vi "initialize StrainCell.vi"(9 "字符串":string, 11 "config in":T1={"initialize"=enum."SR830", "6221"={"6221 Resource"="GPIB1::10::INSTR", "Delta status"=FALSE, "电流|RMS(A)"=0.0}, "SR830+6221"={"source"=0, "Current(A)"=0.0, "阻抗(Ohm)"=0.0, "SR830 1"=FALSE, "SR830 2"=FALSE, "SR830 3"=FALSE, "SR830 4"=FALSE, "VISA 1"="GPIB1::1::INSTR", "VISA 2"="GPIB1::2::INSTR", "VISA 3"="GPIB1::3::INSTR", "VISA 4"="GPIB1::4::INSTR", "Reserve 1"=-1, "Reserve 2"=-1, "Reserve 3"=-1, "Reserve 4"=-1, "Sensitivity 1"=-1, "Sensitivity 2"=0, "Sensitivity 3"=-1, "Sensitivity 4"=-1, "量程入 1"=0, "量程入 2"=0, "量程入 3"=0, "量程入 4"=0}, "2400"={"2400"=FALSE, "VISA"="GPIB0::9::INSTR", "Output Level (0)"=1e-05, "Compliance  Level (0.1)"=10.0, "ch"=[1, 2, 1, 2]}, "ch"={"ch"=[], "current"=[], "change?"=[], "holding current\nwhen change ch?"=TRUE, "current offset"=[]}, "Instrument"={"limit"={"Field limit"=0.0, "Field rate limit"=0.0, "Temp limit"=0.0, "Temp low limit"=0.0, "Temp rate limit "=0.0}, "genarl"={"行数"=refnum, "编辑列表框？"=refnum, "列表框"=refnum, "camg 振荡状态"=refnum, "Aborting"=refnum, "数据文件"=refnum, "warning"=refnum, "vi路径"="", "Instrument Type"=enum."PPMS"}, "cmag"={"TM620"="TCPIP0::192.168.1.5::4266::SOCKET", "M24C Resource"="", "4G supply"="", "Temp Status 24C"=refnum, "Temp"=refnum, "9T信号"=refnum, "4g supply status"=refnum, "in-plane"="", "out-plane"="", "in-plane signal"=FALSE, "out-plane signal"=FALSE, "in plane 信号"=refnum, "pzt volt"=refnum, "camg Rate"=refnum}, "lengtou2"={"750 visa"="", "750 rotate"="", "semaphore 340"=refnum, "semaphore 750"=refnum, "750 field status"=refnum, "Input (0:A) 340"=0, "340 Resource"="GPIB0::14::INSTR", "340 Status"=refnum, "Input (0:B) 340"=0, "Loop (0: 1)"=0, "Loop (1: 1)"=0, "TCP master instance"=refnum}, "lengtou"={"TCP master instance"=refnum, "335 Status"=refnum, "335 Resource "="", "Input (0:A) 335"=0, "Input (0:B) 335"=0, "Heater Output (1:1) 335"=0, "semaphore 335"=refnum}, "325 for test"={"quantum design"=refnum, "semaphore 325"=refnum, "325 Resource "="", "Input (0:A) 325"=0, "Heater Output (1:1) 325"=0, "325 Status"=refnum}}, "2614B"={"2614B chA"=FALSE, "2614B chB"=FALSE, "VISA"="GPIB1::5::INSTR"}, "33522b"={"33522b resource name"="GPIB0::16::INSTR", "零电压"=0.0, "最大电压"=150.0, "间隔"=4.0, "最小电压"=-50.0, "loop"=2.0, "压电陶瓷电压(Vpp)"=0.0}, "gating type"=enum."2614(daul)", "层数"=0, "行数"=0, "是否处理"=[], "current 2"=[], "StrainCell"={"RP100 resource name"="GPIB0::16::INSTR", "E4980 resource name"="GPIB0::16::INSTR", "RP100 Reset ?(True)"=TRUE, "Voltage1(V)"=0.0, "Voltage2(V)"=0.0, "interval"=4.0, "slew(V/s)"=1.0}} {"Instrument"."325 for test"."Heater Output (1:1) 325" items=["1"=1, "2"=2]; "Instrument"."325 for test"."Input (0:A) 325" items=["A", "B"]; "Instrument"."lengtou"."Heater Output (1:1) 335" items=["1"=1, "2"=2]; "Instrument"."lengtou"."Input (0:B) 335" items=["A", "B"]; "Instrument"."lengtou"."Input (0:A) 335" items=["A", "B"]; "Instrument"."lengtou2"."Loop (1: 1)" items=["1", "2"]; "Instrument"."lengtou2"."Loop (0: 1)" items=["1", "2"]; "Instrument"."lengtou2"."Input (0:B) 340" items=["A", "B", "C", "D"]; "Instrument"."lengtou2"."Input (0:A) 340" items=["A", "B", "C", "D"]; "SR830+6221"."Sensitivity 4" items=["Auto Gain"=-1, "2 nV/fA"=0, "5 nV/fA"=1, "10 nV/fA"=2, "20 nV/fA"=3, "50 nV/fA"=4, "100 nV/fA"=5, "200 nV/fA"=6, "500 nV/fA"=7, "1 uV/pA"=8, "2 uV/pA"=9, "5 uV/pA"=10, "10 uV/pA"=11, "20 uV/pA"=12, "50 uV/pA"=13, "100 uV/pA"=14, "200 uV/pA"=15, "500 uV/pA"=16, "1 mV/nA"=17, "2 mV/nA"=18, "5 mV/nA"=19, "10 mV/nA"=20, "20 mV/nA"=21, "50 mV/nA"=22, "100 mV/nA"=23, "200 mV/nA"=24, "500 mV/mA"=25, "1 V/uA"=26]; "SR830+6221"."Sensitivity 3" items=["Auto Gain"=-1, "2 nV/fA"=0, "5 nV/fA"=1, "10 nV/fA"=2, "20 nV/fA"=3, "50 nV/fA"=4, "100 nV/fA"=5, "200 nV/fA"=6, "500 nV/fA"=7, "1 uV/pA"=8, "2 uV/pA"=9, "5 uV/pA"=10, "10 uV/pA"=11, "20 uV/pA"=12, "50 uV/pA"=13, "100 uV/pA"=14, "200 uV/pA"=15, "500 uV/pA"=16, "1 mV/nA"=17, "2 mV/nA"=18, "5 mV/nA"=19, "10 mV/nA"=20, "20 mV/nA"=21, "50 mV/nA"=22, "100 mV/nA"=23, "200 mV/nA"=24, "500 mV/mA"=25, "1 V/uA"=26]; "SR830+6221"."Sensitivity 1" items=["Auto Gain"=-1, "2 nV/fA"=0, "5 nV/fA"=1, "10 nV/fA"=2, "20 nV/fA"=3, "50 nV/fA"=4, "100 nV/fA"=5, "200 nV/fA"=6, "500 nV/fA"=7, "1 uV/pA"=8, "2 uV/pA"=9, "5 uV/pA"=10, "10 uV/pA"=11, "20 uV/pA"=12, "50 uV/pA"=13, "100 uV/pA"=14, "200 uV/pA"=15, "500 uV/pA"=16, "1 mV/nA"=17, "2 mV/nA"=18, "5 mV/nA"=19, "10 mV/nA"=20, "20 mV/nA"=21, "50 mV/nA"=22, "100 mV/nA"=23, "200 mV/nA"=24, "500 mV/mA"=25, "1 V/uA"=26]; "SR830+6221"."Sensitivity 2" items=["Auto Gain"=-1, "2 nV/fA"=0, "5 nV/fA"=1, "10 nV/fA"=2, "20 nV/fA"=3, "50 nV/fA"=4, "100 nV/fA"=5, "200 nV/fA"=6, "500 nV/fA"=7, "1 uV/pA"=8, "2 uV/pA"=9, "5 uV/pA"=10, "10 uV/pA"=11, "20 uV/pA"=12, "50 uV/pA"=13, "100 uV/pA"=14, "200 uV/pA"=15, "500 uV/pA"=16, "1 mV/nA"=17, "2 mV/nA"=18, "5 mV/nA"=19, "10 mV/nA"=20, "20 mV/nA"=21, "50 mV/nA"=22, "100 mV/nA"=23, "200 mV/nA"=24, "500 mV/mA"=25, "1 V/uA"=26]; "SR830+6221"."Reserve 4" items=["Auto Reserve"=-1, "High Reserve"=0, "Normal"=1, "Low Noise"=2]; "SR830+6221"."Reserve 3" items=["Auto Reserve"=-1, "High Reserve"=0, "Normal"=1, "Low Noise"=2]; "SR830+6221"."Reserve 2" items=["Auto Reserve"=-1, "High Reserve"=0, "Normal"=1, "Low Noise"=2]; "SR830+6221"."Reserve 1" items=["Auto Reserve"=-1, "High Reserve"=0, "Normal"=1, "Low Noise"=2]; "SR830+6221"."source" items=["SR830 1", "SR830 2", "SR830 3", "SR830 4"]}) -> (3 "输出簇":T1={"initialize"=enum."SR830", "6221"={"6221 Resource"="GPIB0::24::INSTR", "Delta status"=FALSE, "电流|RMS(A)"=0.0}, "SR830+6221"={"source"=0, "Current(A)"=0.0, "阻抗(Ohm)"=0.0, "SR830 1"=FALSE, "SR830 2"=FALSE, "SR830 3"=FALSE, "SR830 4"=FALSE, "VISA 1"="", "VISA 2"="", "VISA 3"="", "VISA 4"="", "Reserve 1"=-1, "Reserve 2"=-1, "Reserve 3"=-1, "Reserve 4"=-1, "Sensitivity 1"=-1, "Sensitivity 2"=-1, "Sensitivity 3"=-1, "Sensitivity 4"=-1, "量程入 1"=0, "量程入 2"=0, "量程入 3"=0, "量程入 4"=0}, "2400"={"2400"=FALSE, "VISA"="GPIB0::9::INSTR", "Output Level (0)"=1e-05, "Compliance  Level (0.1)"=10.0, "ch"=[]}, "ch"={"ch"=[], "current"=[], "change?"=[], "holding current\nwhen change ch?"=FALSE, "current offset"=[]}, "Instrument"={"limit"={"Field limit"=0.0, "Field rate limit"=0.0, "Temp limit"=0.0, "Temp low limit"=0.0, "Temp rate limit "=0.0}, "genarl"={"行数"=refnum, "编辑列表框？"=refnum, "列表框"=refnum, "camg 振荡状态"=refnum, "Aborting"=refnum, "数据文件"=refnum, "warning"=refnum, "vi路径"="", "Instrument Type"=enum."SVSM"}, "cmag"={"TM620"="GPIB0::24::INSTR", "M24C Resource"="GPIB0::24::INSTR", "4G supply"="GPIB0::24::INSTR", "Temp Status 24C"=refnum, "Temp"=refnum, "9T信号"=refnum, "4g supply status"=refnum, "in-plane"="", "out-plane"="", "in-plane signal"=TRUE, "out-plane signal"=FALSE, "in plane 信号"=refnum, "pzt volt"=refnum, "camg Rate"=refnum}, "lengtou2"={"750 visa"="", "750 rotate"="", "semaphore 340"=refnum, "semaphore 750"=refnum, "750 field status"=refnum, "Input (0:A) 340"=1, "340 Resource"="GPIB0::14::INSTR", "340 Status"=refnum, "Input (0:B) 340"=0, "Loop (0: 1)"=1, "Loop (1: 1)"=0, "TCP master instance"=refnum}, "lengtou"={"TCP master instance"=refnum, "335 Status"=refnum, "335 Resource "="GPIB0::24::INSTR", "Input (0:A) 335"=0, "Input (0:B) 335"=0, "Heater Output (1:1) 335"=0, "semaphore 335"=refnum}, "325 for test"={"quantum design"=refnum, "semaphore 325"=refnum, "325 Resource "="GPIB0::13::INSTR", "Input (0:A) 325"=1000, "Heater Output (1:1) 325"=1, "325 Status"=refnum}}, "2614B"={"2614B chA"=FALSE, "2614B chB"=FALSE, "VISA"=""}, "33522b"={"33522b resource name"="GPIB0::16::INSTR", "零电压"=0.0, "最大电压"=148.0, "间隔"=4.0, "最小电压"=-48.0, "loop"=3.0, "压电陶瓷电压(Vpp)"=0.0}, "gating type"=enum."2614(daul)", "层数"=0, "行数"=0, "是否处理"=[], "current 2"=[], "StrainCell"={"RP100 resource name"="GPIB0::16::INSTR", "E4980 resource name"="GPIB0::16::INSTR", "RP100 Reset ?(True)"=TRUE, "Voltage1(V)"=0.0, "Voltage2(V)"=148.0, "interval"=4.0, "slew(V/s)"=-48.0}} {"Instrument"."325 for test"."Heater Output (1:1) 325" items=["1"=1, "2"=2]; "Instrument"."325 for test"."Input (0:A) 325" items=["A", "B"]; "Instrument"."lengtou"."Heater Output (1:1) 335" items=["1"=1, "2"=2]; "Instrument"."lengtou"."Input (0:B) 335" items=["A", "B"]; "Instrument"."lengtou"."Input (0:A) 335" items=["A", "B"]; "Instrument"."lengtou2"."Loop (1: 1)" items=["1", "2"]; "Instrument"."lengtou2"."Loop (0: 1)" items=["1", "2"]; "Instrument"."lengtou2"."Input (0:B) 340" items=["A", "B", "C", "D"]; "Instrument"."lengtou2"."Input (0:A) 340" items=["A", "B", "C", "D"]; "SR830+6221"."Sensitivity 4" items=["Auto Gain"=-1, "2 nV/fA"=0, "5 nV/fA"=1, "10 nV/fA"=2, "20 nV/fA"=3, "50 nV/fA"=4, "100 nV/fA"=5, "200 nV/fA"=6, "500 nV/fA"=7, "1 uV/pA"=8, "2 uV/pA"=9, "5 uV/pA"=10, "10 uV/pA"=11, "20 uV/pA"=12, "50 uV/pA"=13, "100 uV/pA"=14, "200 uV/pA"=15, "500 uV/pA"=16, "1 mV/nA"=17, "2 mV/nA"=18, "5 mV/nA"=19, "10 mV/nA"=20, "20 mV/nA"=21, "50 mV/nA"=22, "100 mV/nA"=23, "200 mV/nA"=24, "500 mV/mA"=25, "1 V/uA"=26]; "SR830+6221"."Sensitivity 3" items=["Auto Gain"=-1, "2 nV/fA"=0, "5 nV/fA"=1, "10 nV/fA"=2, "20 nV/fA"=3, "50 nV/fA"=4, "100 nV/fA"=5, "200 nV/fA"=6, "500 nV/fA"=7, "1 uV/pA"=8, "2 uV/pA"=9, "5 uV/pA"=10, "10 uV/pA"=11, "20 uV/pA"=12, "50 uV/pA"=13, "100 uV/pA"=14, "200 uV/pA"=15, "500 uV/pA"=16, "1 mV/nA"=17, "2 mV/nA"=18, "5 mV/nA"=19, "10 mV/nA"=20, "20 mV/nA"=21, "50 mV/nA"=22, "100 mV/nA"=23, "200 mV/nA"=24, "500 mV/mA"=25, "1 V/uA"=26]; "SR830+6221"."Sensitivity 1" items=["Auto Gain"=-1, "2 nV/fA"=0, "5 nV/fA"=1, "10 nV/fA"=2, "20 nV/fA"=3, "50 nV/fA"=4, "100 nV/fA"=5, "200 nV/fA"=6, "500 nV/fA"=7, "1 uV/pA"=8, "2 uV/pA"=9, "5 uV/pA"=10, "10 uV/pA"=11, "20 uV/pA"=12, "50 uV/pA"=13, "100 uV/pA"=14, "200 uV/pA"=15, "500 uV/pA"=16, "1 mV/nA"=17, "2 mV/nA"=18, "5 mV/nA"=19, "10 mV/nA"=20, "20 mV/nA"=21, "50 mV/nA"=22, "100 mV/nA"=23, "200 mV/nA"=24, "500 mV/mA"=25, "1 V/uA"=26]; "SR830+6221"."Sensitivity 2" items=["Auto Gain"=-1, "2 nV/fA"=0, "5 nV/fA"=1, "10 nV/fA"=2, "20 nV/fA"=3, "50 nV/fA"=4, "100 nV/fA"=5, "200 nV/fA"=6, "500 nV/fA"=7, "1 uV/pA"=8, "2 uV/pA"=9, "5 uV/pA"=10, "10 uV/pA"=11, "20 uV/pA"=12, "50 uV/pA"=13, "100 uV/pA"=14, "200 uV/pA"=15, "500 uV/pA"=16, "1 mV/nA"=17, "2 mV/nA"=18, "5 mV/nA"=19, "10 mV/nA"=20, "20 mV/nA"=21, "50 mV/nA"=22, "100 mV/nA"=23, "200 mV/nA"=24, "500 mV/mA"=25, "1 V/uA"=26]; "SR830+6221"."Reserve 4" items=["Auto Reserve"=-1, "High Reserve"=0, "Normal"=1, "Low Noise"=2]; "SR830+6221"."Reserve 3" items=["Auto Reserve"=-1, "High Reserve"=0, "Normal"=1, "Low Noise"=2]; "SR830+6221"."Reserve 2" items=["Auto Reserve"=-1, "High Reserve"=0, "Normal"=1, "Low Noise"=2]; "SR830+6221"."Reserve 1" items=["Auto Reserve"=-1, "High Reserve"=0, "Normal"=1, "Low Noise"=2]; "SR830+6221"."source" items=["SR830 1", "SR830 2", "SR830 3", "SR830 4"]})   [LabVIEW 2019, in "nematic.lvlib" / "Copy of StrainCell.lvlib"]
uses:
  nematic/Copy of StrainCell.lvlib
  ctl/config.ctl
  <vilib>/NI/Modbus Library/API/Master/Modbus Master.lvclass
  ctl/initialize.ctl
  ctl/Instrument.ctl
  ctl/limit.ctl
  ctl/warning.ctl
  ctl/Instrument Type.ctl
  ctl/335 state.ctl
  ctl/9T mag field stauts.ctl
  C:/Users/fuyang/Desktop/postdoctor/labview/labview-measure/lib/QDInstrument.dll
  lib/QDInstrument.dll
  ctl/Gating type.ctl
  lib/Keithley 622x/Configure/2182 -A/Low Level/Typedefs/KE2182 -- Voltage Ranges.ctl
  lib/Keithley 622x/Configure/2182 -A/Low Level/Typedefs/KE2182 -- Filter Type.ctl
  lib/Keithley 622x/Configure/2182 -A/Low Level/Typedefs/KE2182 -- Filter Count.ctl
  lib/Keithley 622x/Configure/2182 -A/Low Level/Typedefs/KE2182 -- Filter Window.ctl
  lib/Keithley 622x/Configure/2182 -A/Low Level/Typedefs/KE2182 -- NPLCs.ctl
  lib/Keithley 622x/Configure/Delta PDelta DCon Modes/Typedefs/KE622x -- Delta Mode Params.ctl
  lib/Keithley 622x/Configure/Delta PDelta DCon Modes/Low Level/Typedefs/KE622x -- Delta PDelta Mode High Level.ctl
  lib/Keithley 622x/Configure/Delta PDelta DCon Modes/Low Level/Typedefs/KE622x -- Delta PDelta Mode Low Level.ctl
  lib/Keithley 622x/Configure/Delta PDelta DCon Modes/Low Level/Typedefs/KE622x -- Delta DCon Mode Delay.ctl
  lib/Keithley 622x/Configure/Delta PDelta DCon Modes/Low Level/Typedefs/KE622x -- Delta PDelta Mode Num Cycles Mode.ctl
  lib/Keithley 622x/Configure/Delta PDelta DCon Modes/Low Level/Typedefs/KE622x -- Delta PDelta Mode Num Cycles.ctl
  lib/Keithley 622x/Configure/Source/Typedefs/KE622x -- Voltage Limit.ctl
  lib/Keithley 622x/Configure/Units/Typedefs/KE622x -- Voltage Meas Units.ctl
  lib/Agilent E4980/Agilent E4980.lvlib
  lib/RP100/RP100.lvlib
  lib/Keithley 622x/Keithley 622x.lvlib
panel:
  in  "RP100 Reset ?(True)":bool
  in  "Voltage Limit (V)":T8=10.0 min=0.1 max=105.0 step=0.01 format="%.2p"
  in  "Delta Mode Params In":T9={"High Level (A)"=0.001, "Low Level (A)"=-0.001, "Delay (s)"=0.002, "Num Cycles Mode"=enum."Finite Count", "Finite Count"=1, "Abort On\nCompliance?"=FALSE, "Cold Swithing\nMode Enabled?"=FALSE} {"Finite Count" min=1 max=65536; "Low Level (A)" min=-0.105 max=0.0 format="%.3p"; "High Level (A)" min=0.0 max=0.105 format="%.3p"; "Delay (s)" min=0.001 max=9999.999 format="%.3f"}
  in  "2812 -A Params In":T20={"Auto Range?"=FALSE, "Man / Selected\nRange"=enum."10mV", "Enable Digital\nFilter?"=FALSE, "Filter Type"=enum."Moving", "Filter Count"=10, "Filter\nWindow (%)"=0.01, "Enable Analog\nFilter?"=FALSE, "NPLCs"=5} {"Filter\nWindow (%)" min=0.0 max=10.0 step=0.01 format="%.2f"; "Filter Count" min=1 max=100; "NPLCs" min=1 max=10}
  out "error out":errorcluster
  in  "error in (no error)":errorcluster
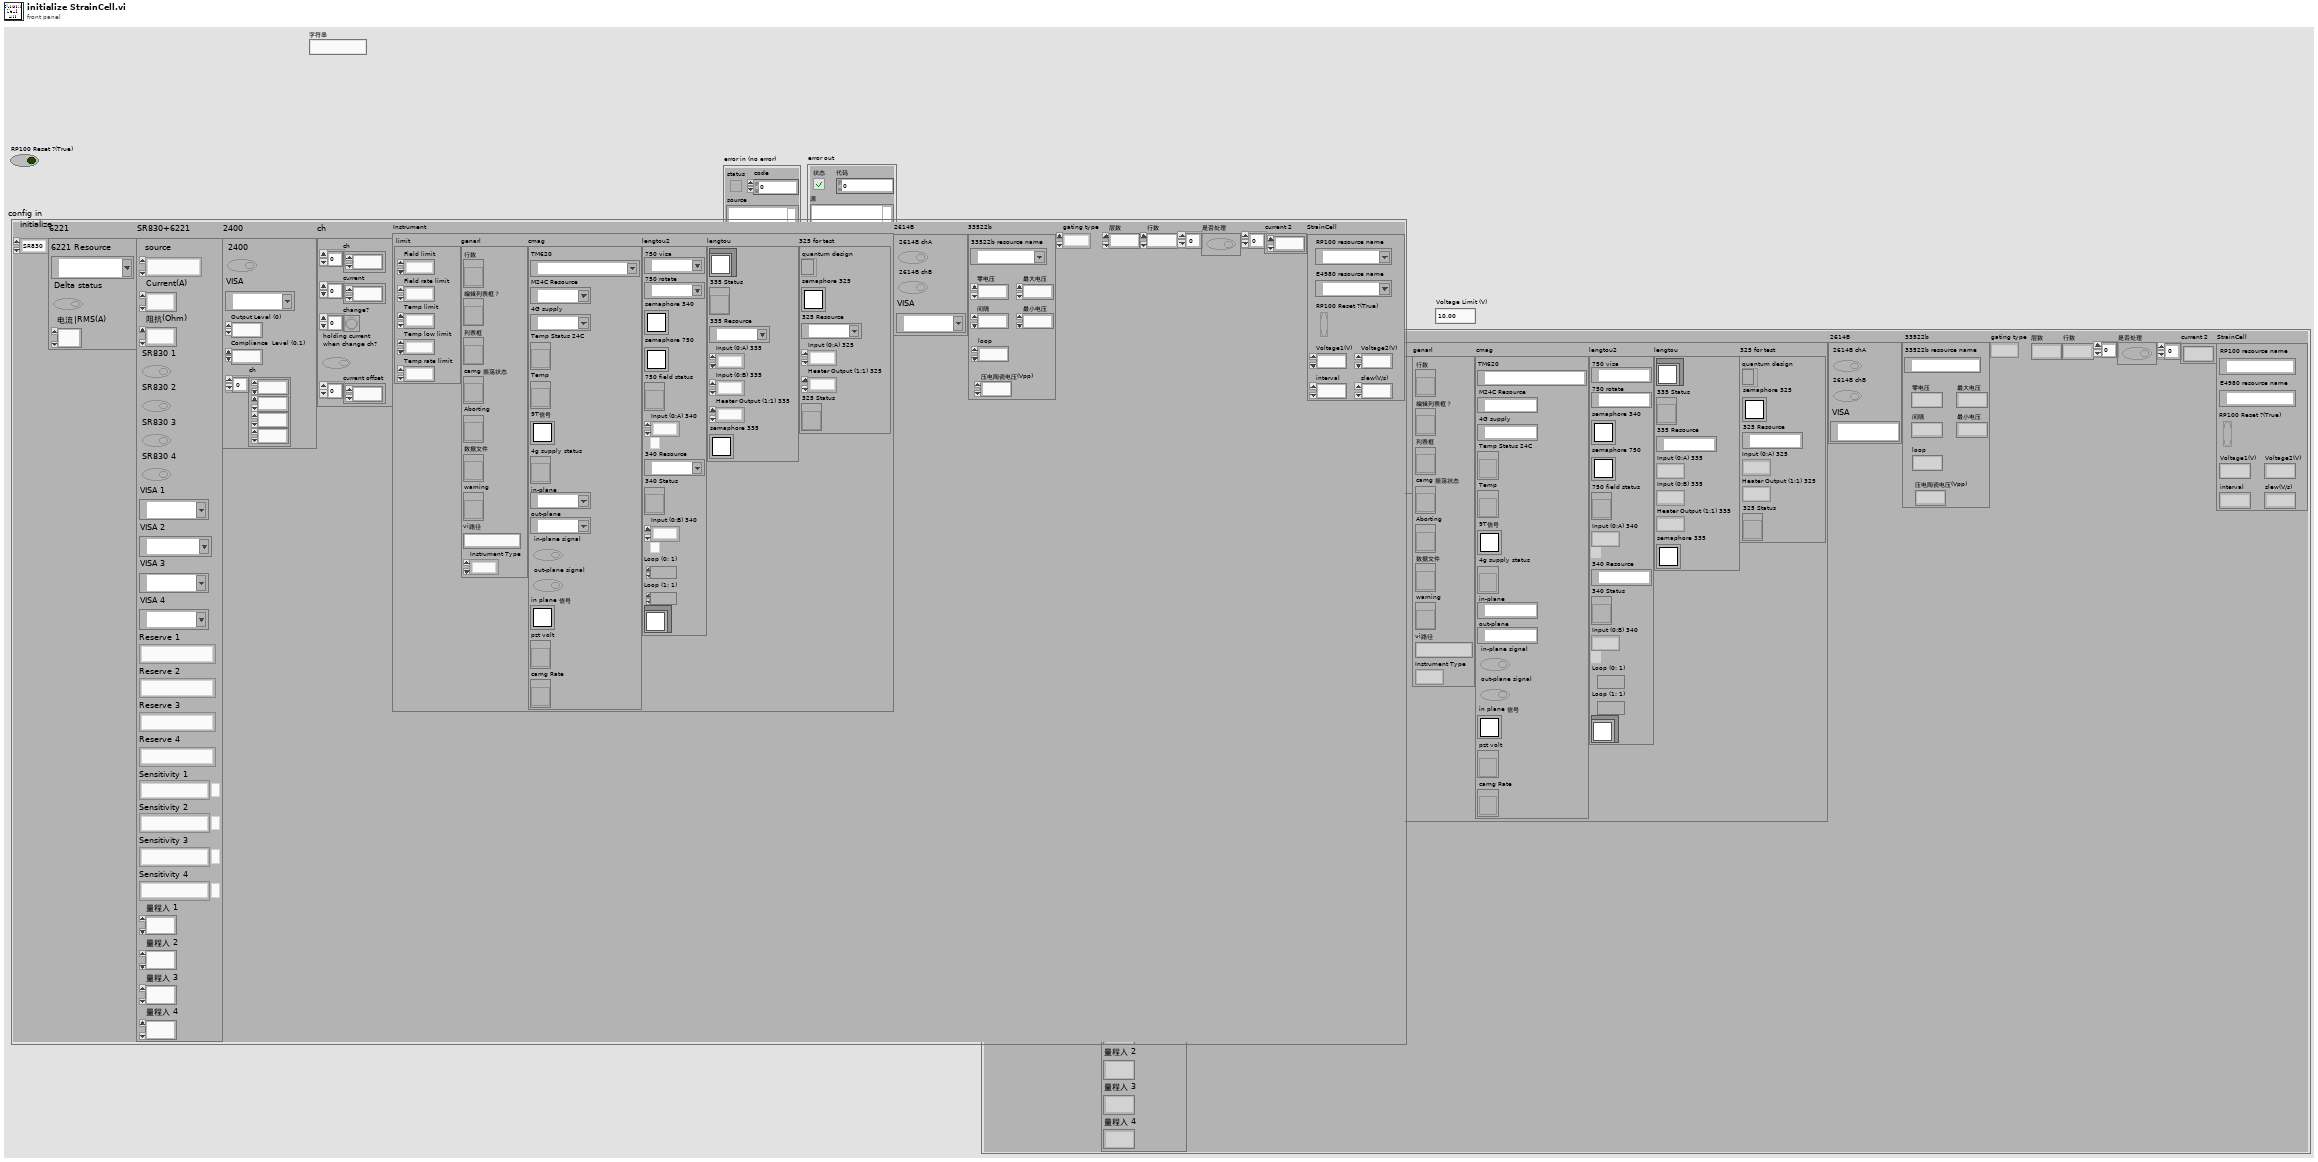
[diagram p1: front panel]
types:
  T1 = typedef "config.ctl" = cluster{"initialize":T2, "6221":cluster{"6221 Resource":refnum<visa-resource-name>, "Delta status":bool, "电流|RMS(A)":dbl}, "SR830+6221":cluster{"source":u16, "Current(A)":dbl, "阻抗(Ohm)":dbl, "SR830 1":bool, "SR830 2":bool, "SR830 3":bool, "SR830 4":bool, "VISA 1":refnum<visa-resource-name>, "VISA 2":refnum<visa-resource-name>, "VISA 3":refnum<visa-resource-name>, "VISA 4":refnum<visa-resource-name>, "Reserve 1":i16, "Reserve 2":i16, "Reserve 3":i16, "Reserve 4":i16, "Sensitivity 1":i16, "Sensitivity 2":i16, "Sensitivity 3":i16, "Sensitivity 4":i16, "量程入 1":i32, "量程入 2":i32, "量程入 3":i32, "量程入 4":i32}, "2400":cluster{"2400":bool, "VISA":refnum<visa-resource-name>, "Output Level (0)":dbl, "Compliance  Level (0.1)":dbl, "ch":i32[]}, "ch":cluster{"ch":i32[], "current":dbl[], "change?":bool[], "holding current\nwhen change ch?":bool, "current offset":dbl[]}, "Instrument":T3, "2614B":cluster{"2614B chA":bool, "2614B chB":bool, "VISA":refnum<visa-resource-name>}, "33522b":cluster{"33522b resource name":refnum<visa-resource-name>, "零电压":dbl, "最大电压":dbl, "间隔":dbl, "最小电压":dbl, "loop":dbl, "压电陶瓷电压(Vpp)":dbl}, "gating type":T7, "层数":i32, "行数":i32, "是否处理":bool[], "current 2":dbl[], "StrainCell":cluster{"RP100 resource name":refnum<visa-resource-name>, "E4980 resource name":refnum<visa-resource-name>, "RP100 Reset ?(True)":bool, "Voltage1(V)":dbl, "Voltage2(V)":dbl, "interval":dbl, "slew(V/s)":dbl}}
  T2 = typedef "initialize.ctl" = enum16{"SR830", "keithley6221-SR830", "Delta", "Delta-tunnelling", "keithley6221-2182-DC", "PZT", "StrainCell", "4200"}
  T3 = typedef "Instrument.ctl" = cluster{"limit":T4, "genarl":cluster{"行数":refnum<vi>, "编辑列表框？":refnum<vi>, "列表框":refnum<vi>, "camg 振荡状态":refnum<vi>, "Aborting":refnum<vi>, "数据文件":refnum<vi>, "warning":refnum<vi>, "vi路径":string, "Instrument Type":T5}, "cmag":cluster{"TM620":refnum<visa-resource-name>, "M24C Resource":refnum<visa-resource-name>, "4G supply":refnum<visa-resource-name>, "Temp Status 24C":refnum<vi>, "Temp":refnum<vi>, "9T信号":T6, "4g supply status":refnum<vi>, "in-plane":refnum<visa-resource-name>, "out-plane":refnum<visa-resource-name>, "in-plane signal":bool, "out-plane signal":bool, "in plane 信号":T6, "pzt volt":refnum<vi>, "camg Rate":refnum<vi>}, "lengtou2":cluster{"750 visa":refnum<visa-resource-name>, "750 rotate":refnum<visa-resource-name>, "semaphore 340":T6, "semaphore 750":T6, "750 field status":refnum<vi>, "Input (0:A) 340":u16, "340 Resource":refnum<visa-resource-name>, "340 Status":refnum<vi>, "Input (0:B) 340":u16, "Loop (0: 1)":u16, "Loop (1: 1)":u16, "TCP master instance":refnum<class "Modbus Master.lvclass">}, "lengtou":cluster{"TCP master instance":refnum<class "Modbus Master.lvclass">, "335 Status":refnum<vi>, "335 Resource ":refnum<visa-resource-name>, "Input (0:A) 335":u16, "Input (0:B) 335":u16, "Heater Output (1:1) 335":u16, "semaphore 335":T6}, "325 for test":cluster{"quantum design":refnum<k24>, "semaphore 325":T6, "325 Resource ":refnum<visa-resource-name>, "Input (0:A) 325":u16, "Heater Output (1:1) 325":u16, "325 Status":refnum<vi>}}
  T4 = typedef "limit.ctl" = cluster{"Field limit":dbl, "Field rate limit":dbl, "Temp limit":dbl, "Temp low limit":dbl, "Temp rate limit ":dbl}
  T5 = typedef "Instrument Type.ctl" = enum16{"PPMS", "VersaLab", "DynaCool", "SVSM", "PPMS-Rotate", "Lakeshore335", "2T cmag", "9T mag old", "9T cmag", "9T cmag DAC", "9T cmag rotate", "test"}
  T6 = typedef "Semaphore RefNum" = refnum<k1>
  T7 = typedef "Gating type.ctl" = enum32{"null", "2614(daul)", "2400", "6517B"}
  T8 = typedef "Keithley 622x.lvlib/KE622x -- Voltage Limit.ctl" = dbl
  T9 = typedef "Keithley 622x.lvlib/KE622x -- Delta Mode Params.ctl" = cluster{"High Level (A)":T10, "Low Level (A)":T11, "Delay (s)":T12, "Num Cycles Mode":T13, "Finite Count":T14, "Abort On\nCompliance?":bool, "Cold Swithing\nMode Enabled?":bool}
  T10 = typedef "Keithley 622x.lvlib/KE622x -- Delta PDelta Mode High Level.ctl" = dbl
  T11 = typedef "Keithley 622x.lvlib/KE622x -- Delta PDelta Mode Low Level.ctl" = dbl
  T12 = typedef "Keithley 622x.lvlib/KE622x -- Delta DCon Mode Delay.ctl" = dbl
  T13 = typedef "Keithley 622x.lvlib/KE622x -- Delta PDelta Mode Num Cycles Mode.ctl" = enum16{"Finite Count", "Infinite"}
  T14 = typedef "Keithley 622x.lvlib/KE622x -- Delta PDelta Mode Num Cycles.ctl" = u32
  T15 = typedef "Keithley 622x.lvlib/KE2182 -- Voltage Ranges.ctl" = enum16{"10mV", "100mV", "1V", "10V", "100V"}
  T16 = typedef "Keithley 622x.lvlib/KE2182 -- Filter Type.ctl" = enum16{"Moving", "Repeat"}
  T17 = typedef "Keithley 622x.lvlib/KE2182 -- Filter Count.ctl" = u32
  T18 = typedef "Keithley 622x.lvlib/KE2182 -- Filter Window.ctl" = dbl
  T19 = typedef "Keithley 622x.lvlib/KE2182 -- NPLCs.ctl" = u32
  T20 = cluster{"Auto Range?":bool, "Man / Selected\nRange":T15, "Enable Digital\nFilter?":bool, "Filter Type":T16, "Filter Count":T17, "Filter\nWindow (%)":T18, "Enable Analog\nFilter?":bool, "NPLCs":T19}
  T21 = typedef "Keithley 622x.lvlib/KE622x -- Voltage Meas Units.ctl" = enum16{"Volts", "Ohms", "Watts", "Siemens"}
  T22 = typedef "Keithley 622x.lvlib/KE622x -- On Off Control.ctl" = enum16{"Off", "On"}
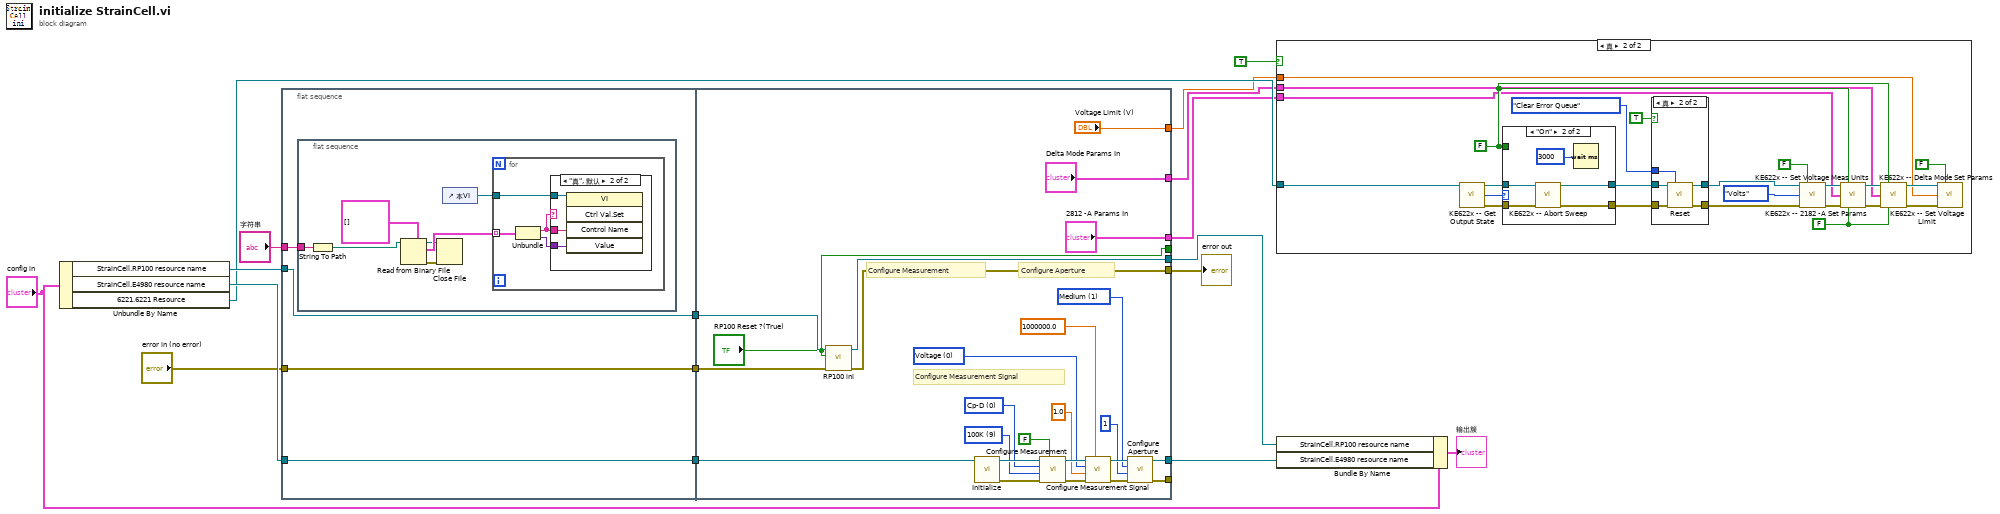
[diagram p0: block diagram]
diagram:
  n1 = Unbundle By Name("config in") -> ("StrainCell.RP100 resource name"=w16:refnum<visa-resource-name>, "StrainCell.E4980 resource name"=w17:refnum<visa-resource-name>, "6221.6221 Resource"=w7:refnum<visa-resource-name>)
  n2 = flat-sequence {
    tunnel: "error in (no error)" -> [w19]
    tunnel: w16 -> [w20]
    tunnel: w17 -> [w21]
    tunnel: [w21] -> w11
    tunnel: [w20] -> w10
    tunnel: [w19] -> w9
    tunnel: "字符串" -> [w18]
    tunnel: [w54] -> w1
    tunnel: [w53] -> _
    tunnel: [w51] -> w15
    tunnel: [w49] -> w12
    tunnel: ["RP100 Reset ?(True)"] -> _
    tunnel: w11 -> [w55]
    tunnel: w10 -> [w52]
    tunnel: w9 -> [w50]
    tunnel: ["Voltage Limit (V)"] -> w5
    tunnel: ["Delta Mode Params In"] -> w4
    tunnel: ["2812 -A Params In"] -> w6
    frame #0 {
      n3 = flat-sequence {
        tunnel: w18 -> [w22]
        frame #0 {
          n4 = String To Path(string=w22) -> (path=w27:path)
          n5 = Read from Binary File(5:cluster{"Name":string, "Variant Data":variant}[] [] ("控件值:获取全部"), 11:w27) -> (0:w23:errorcluster, 2:w25:cluster{"Name":string, "Variant Data":variant}[], 3:w24:refnum<file>)  [unwired: 4 in, 1 out]
          n6 = Close File(refnum=w24, error in=w23) -> ()  [unwired: 2 out]
          n7 = control-ref of="本VI"() -> (w28:refnum<vi>)
          n8 = for {
            tunnel: w25 -> [w32] mode=indexing
            tunnel: w28 -> [w31]
            n9 = Unbundle(w32) -> ("Name"=w29:string, "Variant Data"=w30:variant)
            n10 = case shown="\"真\", 默认" w29 {
              tunnel: w31 -> [_ w35]
              tunnel: w29 -> [_ w34]
              tunnel: w30 -> [_ w33]
              frame "cancel", "load", "model", "ok" {
              }
              frame "真", Default {
                n11 = invoke class="VI" method="Ctrl Val.Set"(reference=w35, "Control Name"=w34, "Value"=w33) -> ()  [unwired: 2 in, 5 out]
              }
            }
          }
        }
      }
    }
    frame #1 {
      w41 = u16 0 items=["Cp-D", "Cp-Q", "Cp-G", "Cp-Rp", "Cs-D", "Cs-Q", "Cs-Rs", "Lp-D", "Lp-Q", "Lp-G", "Lp-Rp", "Lp-Rdc", "Ls-D", "Ls-Q", "Ls-Rs", "Ls-Rdc", "R-X", "Z-thd", "Z-thr", "G-B", "Y-thd", "Y-thr", "Vdc-Idc"] ("Function (0: Cp-D)")
      w44 = u16 1 items=["Short", "Medium", "Long"] ("Measurement Time (1: Medium)")
      w45 = u16 0 items=["Voltage", "Current"] ("Signal Type (0: Voltage)")
      w47 = 9 items=["100m", "1", "10", "100", "300", "1K", "3K", "10K", "30K", "100K"] ("Manual Impedance Range (3: 100 Ohms)")
      # "Configure Aperture"
      # "Configure Measurement Signal"
      # "Configure Measurement"
      n12 = call "RP100 ini.vi"("error in (no error)"=w50, "Reset? (T)"="RP100 Reset ?(True)", "VISA resource name"=w52) -> ("error out"=w49:errorcluster, "VISA resource name out"=w51:refnum<visa-resource-name>)  [unwired: 7 in]
      n13 = call "Initialize.vi"("VISA resource name"=w55) -> ("error out"=w60:errorcluster, "VISA resource name out"=w48:refnum<visa-resource-name>)  [unwired: 9 in]
      n14 = call "Configure Measurement.vi"("Enable Auto Range (T:Enable)"=FALSE, "error in (no error)"=w60, "Manual Impedance Range (3: 100 Ohms)"=w47, "Function (0: Cp-D)"=w41, "VISA resource name"=w48) -> ("error out"=w58:errorcluster, "VISA resource name out"=w59:refnum<visa-resource-name>)  [unwired: 5 in]
      n15 = call "Configure Measurement Signal.vi"("Signal Frequency (1000 Hz)"=1000000.0, "error in (no error)"=w58, "Signal Level (1.0 V)"=1.0, "Signal Type (0: Voltage)"=w45, "VISA resource name"=w59) -> ("error out"=w56:errorcluster, "VISA resource name out"=w57:refnum<visa-resource-name>)  [unwired: 5 in]
      n16 = call "Configure Aperture.vi"("error in (no error)"=w56, "Averaging Factor (1)"=1, "Measurement Time (1: Medium)"=w44, "VISA resource name"=w57) -> ("error out"=w53:errorcluster, "VISA resource name out"=w54:refnum<visa-resource-name>)  [unwired: 6 in]
    }
  }
  n17 = case shown="真" TRUE {
    tunnel: w7 -> [_ w65]
    tunnel: w6 -> [_ w64]
    tunnel: w5 -> [_ w63]
    tunnel: w4 -> [_ w62]
    frame False {
    }
    frame True {
      w80 = FALSE
      w73 = FALSE
      n18 = call "KE622x -- Get Output State.vi"("Resource In"=w65) -> ("Resource Out (dupl)"=w74:refnum<visa-resource-name>, "Output State"=w69:T22, "error out"=w71:errorcluster)  [unwired: 12 in]
      n19 = case shown="\"On\"" w69 {
        tunnel: w74 -> [w86 w90]
        tunnel: w73 -> [_ _]
        tunnel: [w86 w89] -> w72
        tunnel: w71 -> [w85 w88]
        tunnel: [w85 w87] -> w70
        frame "Off", Default {
        }
        frame "On" {
          n20 = call "KE622x -- Abort Sweep.vi"("Resource In"=w90, "error in (no error)"=w88) -> ("Resource Out (dupl)"=w89:refnum<visa-resource-name>, "error out"=w87:errorcluster)  [unwired: 12 in]
          n21 = Wait (ms)(milliseconds to wait=u32 3000 ("等待时间（毫秒）")) -> ()  [unwired: 1 out]
        }
      }
      n22 = case shown="真" TRUE {
        tunnel: w72 -> [w93 w98]
        tunnel: enum16{"Clear Error Queue", "Error Query"}."Clear Error Queue" ("Error Queue Option") -> [_ w97]
        tunnel: [w93 w96] -> w83
        tunnel: w70 -> [w92 w95]
        tunnel: [w92 w94] -> w77
        frame False {
        }
        frame True {
          n23 = call "Reset.vi"("VISA resource name"=w98, "Error Queue Option"=w97, "error in (no error)"=w95) -> ("VISA resource name out"=w96:refnum<visa-resource-name>, "error out"=w94:errorcluster)  [unwired: 11 in]
        }
      }
      n24 = call "KE622x -- Set Voltage Meas Units.vi"("Resource In"=w83, "Check For SCPI Errors? (T)"=FALSE, "Voltage Meas Units"=KE622x_--_Voltage_Meas_Units."Volts", "error in (no error)"=w77) -> ("Resource Out (dupl)"=w84:refnum<visa-resource-name>, "error out"=w76:errorcluster)  [unwired: 10 in]
      n25 = call "KE622x -- 2182 -A Set Params.vi"("622x Resource In"=w84, "Check For SCPI Errors? (T)"=w73, "2812 -A Params In"=w64, "error in (no error)"=w76, "Read Back Set Values? (T)"=w80) -> ("622x Resource Out (dupl)"=w82:refnum<visa-resource-name>, "error out"=w75:errorcluster)  [unwired: 8 in, 1 out]
      n26 = call "KE622x -- Delta Mode Set Params.vi"("Resource In"=w82, "Check For SCPI Errors? (T)"=w73, "Delta Mode Params In"=w62, "error in (no error)"=w75, "Read Back Set Values? (T)"=w80) -> ("Resource Out (dupl)"=w68:refnum<visa-resource-name>, "error out"=w67:errorcluster)  [unwired: 8 in, 1 out]
      n27 = call "KE622x -- Set Voltage Limit.vi"("Resource In"=w68, "Check For SCPI Errors? (T)"=FALSE, "Voltage Limit (V)"=w63, "error in (no error)"=w67) -> ()  [unwired: 10 in, 2 out]
    }
  }
  n28 = Bundle By Name(cluster="config in", "StrainCell.RP100 resource name"=w15, "StrainCell.E4980 resource name"=w1) -> (→"输出簇":T1)
  "error out" <- w12
